vi "Actor Core.vi"(8 "error in":errorcluster, 11 "Automation Controller in":refnum<class "Automation Controller.lvclass">) -> (0 "error out":errorcluster, 3 "Actor out":refnum<class "Actor.lvclass">)   [LabVIEW 2024, in "Automation Controller.lvlib" / "Automation Controller.lvclass"]
doc: "<p>(<strong>Filename</strong>: <span class=\"dnl\">Actor Framework.lvlib:Actor.lvclass:Actor Core.vi</span>)</p>\n<p>Receives messages to the actor, reacts to them, and initiates any error handling that may shut the actor down.</p>\n<p>Descendant classes may override this VI to append parallel tasks for the actor to complete while it handles messages. Overrides use the <a href=\"nihelplauncher://docs/csh?context=lvcore_glang_udclass\">Call Parent Class Method</a> node.</p>"
uses:
  Automation Controller.lvclass
  <vilib>/ActorFramework/Actor/Actor.lvclass
  Idle/Idle/Idle.lvclass
  <vilib>/ActorFramework/Actor/Actor.lvclass/Actor.ctl
  <vilib>/ActorFramework/Message Enqueuer/Message Enqueuer.lvclass/Message Enqueuer.ctl
  Automation Controller Messages/Initial State Msg/Initial State Msg.lvclass/Initial State Msg.ctl
  <vilib>/ActorFramework/Message Enqueuer/Init from Existing Queue.vi
  <vilib>/ActorFramework/Message Enqueuer/Enqueue.vi
  Automation Controller Messages/Initial State Msg/Initial State Msg.lvclass
  <vilib>/ActorFramework/Message Priority Queue/Priority Enqueue.vi
  <vilib>/ActorFramework/Message Enqueuer/Message Enqueuer.lvclass
  State Machine Actor/State Machine Actor/State Machine Actor.lvclass
  Automation Controller.lvclass/Automation Controller.ctl
  C:/Users/uspoaotto/OneDrive - Oregon Tool/Desktop/working copies/stateMachineActor/src/State Machine Actor/State Machine Actor/State Machine Actor.lvclass
  C:/Users/uspoaotto/OneDrive - Oregon Tool/Desktop/working copies/stateMachineActor/src/_State Machine Actor/_State Machine Actor/_State Machine Actor.lvclass
  C:/Program Files (x86)/National Instruments/LabVIEW 2024/vi.lib/ActorFramework/Actor/Actor.lvclass
  C:/Users/uspoaotto/OneDrive - Oregon Tool/Desktop/working copies/stateMachineActor/src/Automation Controller/Automation Controller/Automation Controller.lvclass
  C:/Users/uspoaotto/OneDrive - Oregon Tool/Desktop/working copies/stateMachineActor/src/Idle/Idle/Idle.lvclass
panel:
  out "State Machine Status":T1(array[cluster]) {"Time Stamp" format="%<%x %.2X>T"}
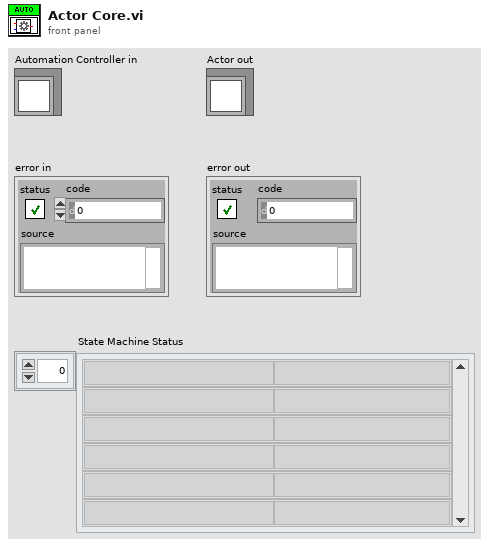
[diagram p1: front panel]
types:
  T1 = cluster{"Time Stamp":timestamp, "String":string}[]
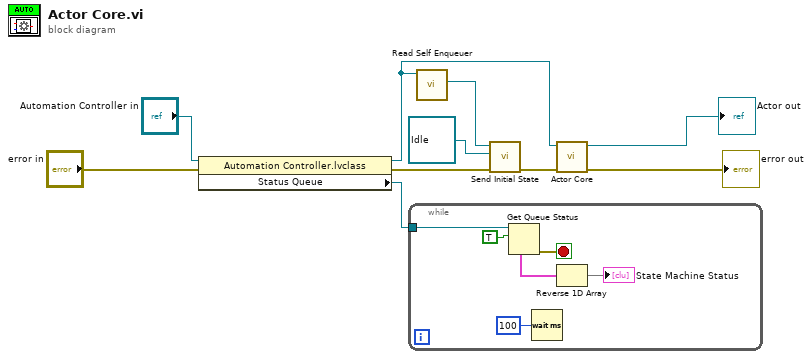
[diagram p0: block diagram]
diagram:
  n1 = property class="Automation Controller.lvclass"(reference="Automation Controller in", error in="error in") -> (reference out=w6:refnum<class "Automation Controller.lvclass">, error out=w1:errorcluster, "Status Queue"=w2:refnum<queue>)
  n2 = while {
    tunnel: w2 -> [w16]
    stop <- w13 stop-if-true
    n3 = Get Queue Status(queue=w16, return elements? (F)=TRUE) -> (error out=w13:errorcluster, elements=w15:cluster{timestamp, string}[])  [unwired: 1 in, 6 out]
    n4 = Wait (ms)(milliseconds to wait=u32 100) -> ()  [unwired: 1 out]
    n5 = Reverse 1D Array(array=w15) -> (reversed array=→"State Machine Status":cluster{timestamp, string}[])
  }
  n6 = call <vilib>:"Read Self Enqueuer.vi"("Actor"=w6) -> ("Self Enqueuer"=w5:refnum<class "Message Enqueuer.lvclass">)  [unwired: 10 in]
  n7 = call "Send Initial State.vi"("error in (no error)"=w1, "Target State in"=refnum<class "Idle.lvclass"> refnum ("Idle.lvlib:Idle.lvclass"), "Message Enqueuer"=w5) -> ("error out"=w3:errorcluster)  [unwired: 7 in, 1 out]
  n8 = call-parent "Actor Core.vi"("error in"=w3, "Actor in"=w6) -> ("error out"=→"error out":errorcluster, "Actor out"=→"Actor out":refnum<class "Actor.lvclass">)  [unwired: 8 in]
